vi "Event Driven Programing.vi"() -> ()   [LabVIEW 2015]
panel:
  out "Waveform Graph":dynamicdata(graph)
  out "Time":timestamp
  out "Tank":dbl(slide) scale=0.0..10.0
  in  "Data Acqusition":bool
  in  "Level":dbl(slide) scale=0.0..10.0
  out "Literas":i32
  in  "Time Check":bool
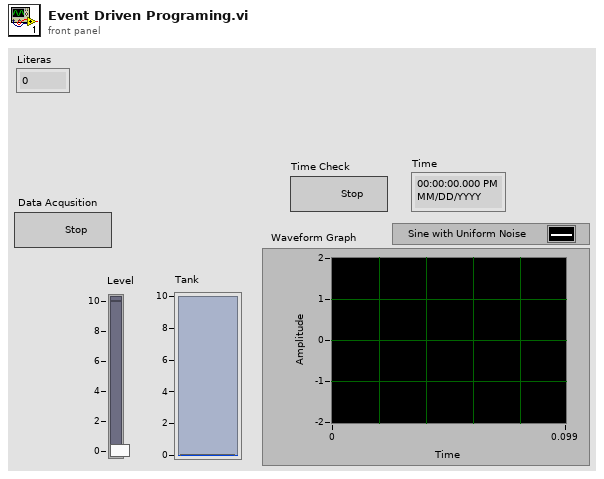
[diagram p1: front panel]
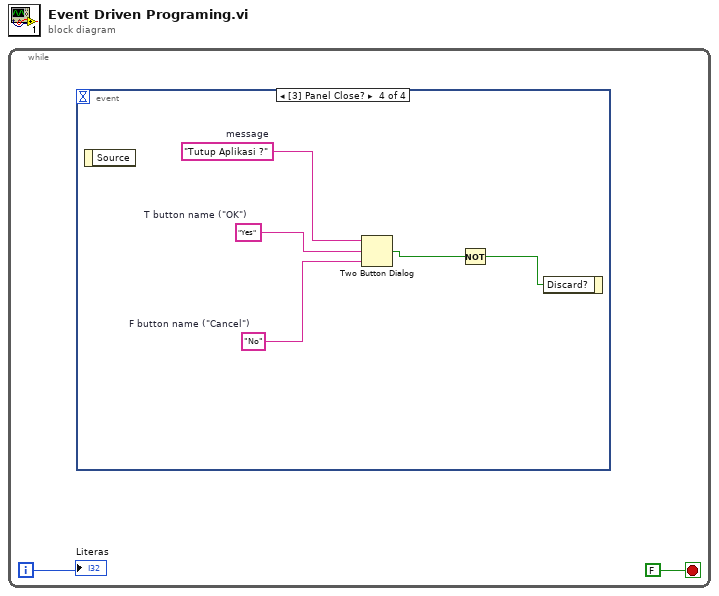
[diagram p0: block diagram]
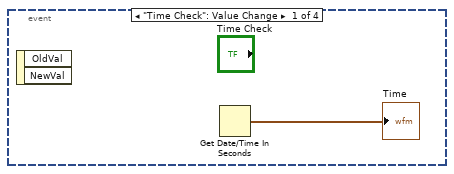
[diagram p2: hidden frame]
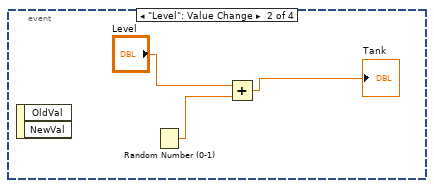
[diagram p3: hidden frame]
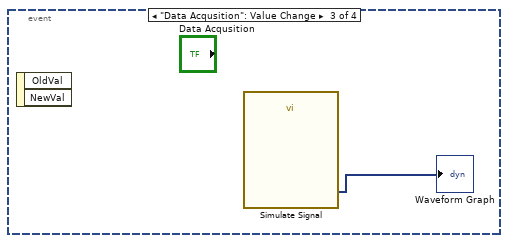
[diagram p4: hidden frame]
diagram:
  n1 = while {
    i -> [w2]
    stop <- FALSE stop-if-true
    n2 = event shown="[3] Panel Close?" {
      selector: _ -> [_ _ _ _]
      dyn-events: _ -> [_ _ _ _]
      timeout: _ -> [_ _ _ _]
      event "Time Check": Value Change {
        n3 = event-data() -> ()  [unwired: 1 in, 2 out]
        n4 = Get Date/Time In Seconds() -> (seconds since 1Jan1904=→"Time":timestamp)
      }
      event "Level": Value Change {
        n5 = event-data() -> ()  [unwired: 1 in, 2 out]
        n6 = Random Number (0-1)() -> (number: 0 to 1=w5:dbl)
        n7 = Add(x="Level", y=w5) -> (x+y=→"Tank":dbl)
      }
      event "Data Acqusition": Value Change {
        n8 = event-data() -> ()  [unwired: 1 in, 2 out]
        n9 = call "Simulate Signal"() -> ("Sine with Uniform Noise"=→"Waveform Graph":dynamicdata)  [unwired: 14 in, 1 out]
      }
      event Panel Close? {
        w10 = "Tutup Aplikasi ?"  # message
        w11 = "No"  # F button name ("Cancel")
        w12 = "Yes"  # T button name ("OK")
        n10 = event-data() -> ()  [unwired: 1 in, 1 out]
        n11 = Two Button Dialog(message=w10, 1:w11, 2:w12) -> (T button?=w9:bool)
        n12 = Not(x=w9) -> (.not. x?=w8:bool)
        n13 = event-data("Discard?"=w8) -> ()  [unwired: 1 in, 1 out]
      }
    }
    "Literas" <- w2
  }
